vi "Start TDMS.vi"(4 "Batch Size":i32, 6 "Thread Count":i32, 8 "error in (no error)":errorcluster, 10 "Path":path, 11 "Application Manager in":refnum<class "Application Manager.lvclass">) -> (0 "error out":errorcluster, 3 "Application Manager out":refnum<class "Application Manager.lvclass">)   [LabVIEW 2025, in "Application Manager.lvlib" / "Application Manager.lvclass"]
uses:
  Application Manager.lvclass
  Application Manager.lvclass/Application Manager.ctl
  TDMS DAQ/TDMS DAQ Messages/Configure TDMS DAQ Msg/Configure TDMS DAQ Msg.lvclass
  DAQ Interface/DAQ Interface Messages/Start DAQ Msg/Start DAQ Msg.lvclass
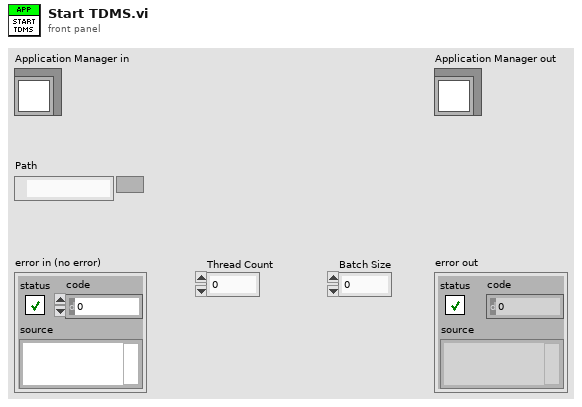
[diagram p1: front panel]
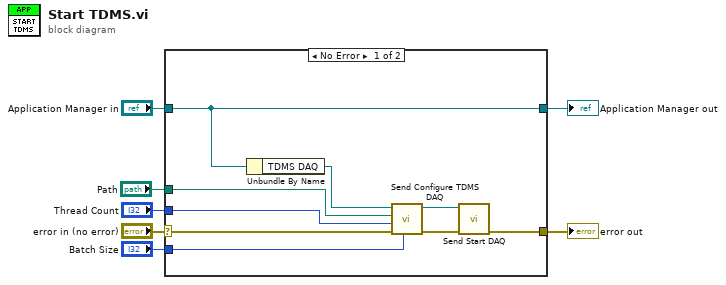
[diagram p0: block diagram]
diagram:
  n1 = case shown="No Error" "error in (no error)" {
    selector: "error in (no error)" -> [w13 w18]
    tunnel: [w8 w18] -> w6
    tunnel: [w16 w17] -> w4
    tunnel: "Application Manager in" -> [w16 w17]
    tunnel: "Path" -> [w11 _]
    tunnel: "Thread Count" -> [w10 _]
    tunnel: "Batch Size" -> [w9 _]
    frame No Error {
      n2 = Unbundle By Name(w16) -> ("TDMS DAQ"=w12:refnum<class "Message Enqueuer.lvclass">)
      n3 = call "Send Configure TDMS DAQ.vi"("Batch Size"=w9, "error in (no error)"=w13, "Thread Count"=w10, "Path"=w11, "Message Enqueuer"=w12) -> ("error out"=w14:errorcluster, "Message Enqueuer out"=w15:refnum<class "Message Enqueuer.lvclass">)  [unwired: 5 in]
      n4 = call "Send Start DAQ.vi"("error in (no error)"=w14, "Message Enqueuer"=w15) -> ("error out"=w8:errorcluster)  [unwired: 8 in, 1 out]
    }
    frame Error {
    }
  }
  "error out" <- w6
  "Application Manager out" <- w4
